vi "InitializeBuffers.vi"(0 "BufferConfig":T1={"Channels"=[], "pretriggerTime_sec"=0.0, "posttriggerTime_sec"=0.0, "BlockSizePerChannel"=0, "SampleRate_Hz"=0.0, "decimation factor"=1, "logDirectory"="", "logPrefix"="", "max files"=0}, 11 "error in (no error)":errorcluster) -> (4 "Buffers":T2={"Channels"=[], "PosttriggerBuffer"=refnum, "PretriggerBuffer"=refnum, "BlockSizePerChannel"=0, " logging semaphore"=refnum, "Log refnum"=refnum, "snapshotBuffer"=refnum, "logDirectory"=path "", "logPrefix"="", "decimation factor"=1, "max files"=0, "SampleRate"=0.0}, 15 "error out":errorcluster)   [LabVIEW 2017, in "BufferLogging.lvlib"]
uses:
  BufferLogging.lvlib
  Buffers.ctl
  BufferConfig.ctl
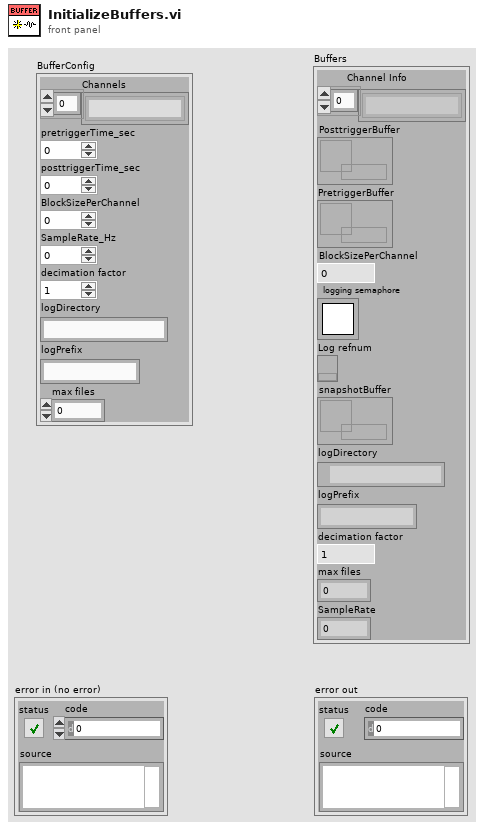
[diagram p1: front panel]
types:
  T1 = typedef "BufferLogging.lvlib/BufferConfig.ctl" = cluster{"Channels":string[], "pretriggerTime_sec":dbl, "posttriggerTime_sec":dbl, "BlockSizePerChannel":i32, "SampleRate_Hz":dbl, "decimation factor":i32, "logDirectory":string, "logPrefix":string, "max files":i32}
  T2 = typedef "BufferLogging.lvlib/Buffers.ctl" = cluster{"Channels":string[], "PosttriggerBuffer":refnum<queue>, "PretriggerBuffer":refnum<queue>, "BlockSizePerChannel":i32, " logging semaphore":T3, "Log refnum":refnum<k34>, "snapshotBuffer":refnum<data-value>, "logDirectory":path, "logPrefix":string, "decimation factor":i32, "max files":i32, "SampleRate":dbl}
  T3 = typedef "Semaphore RefNum" = refnum<k1>
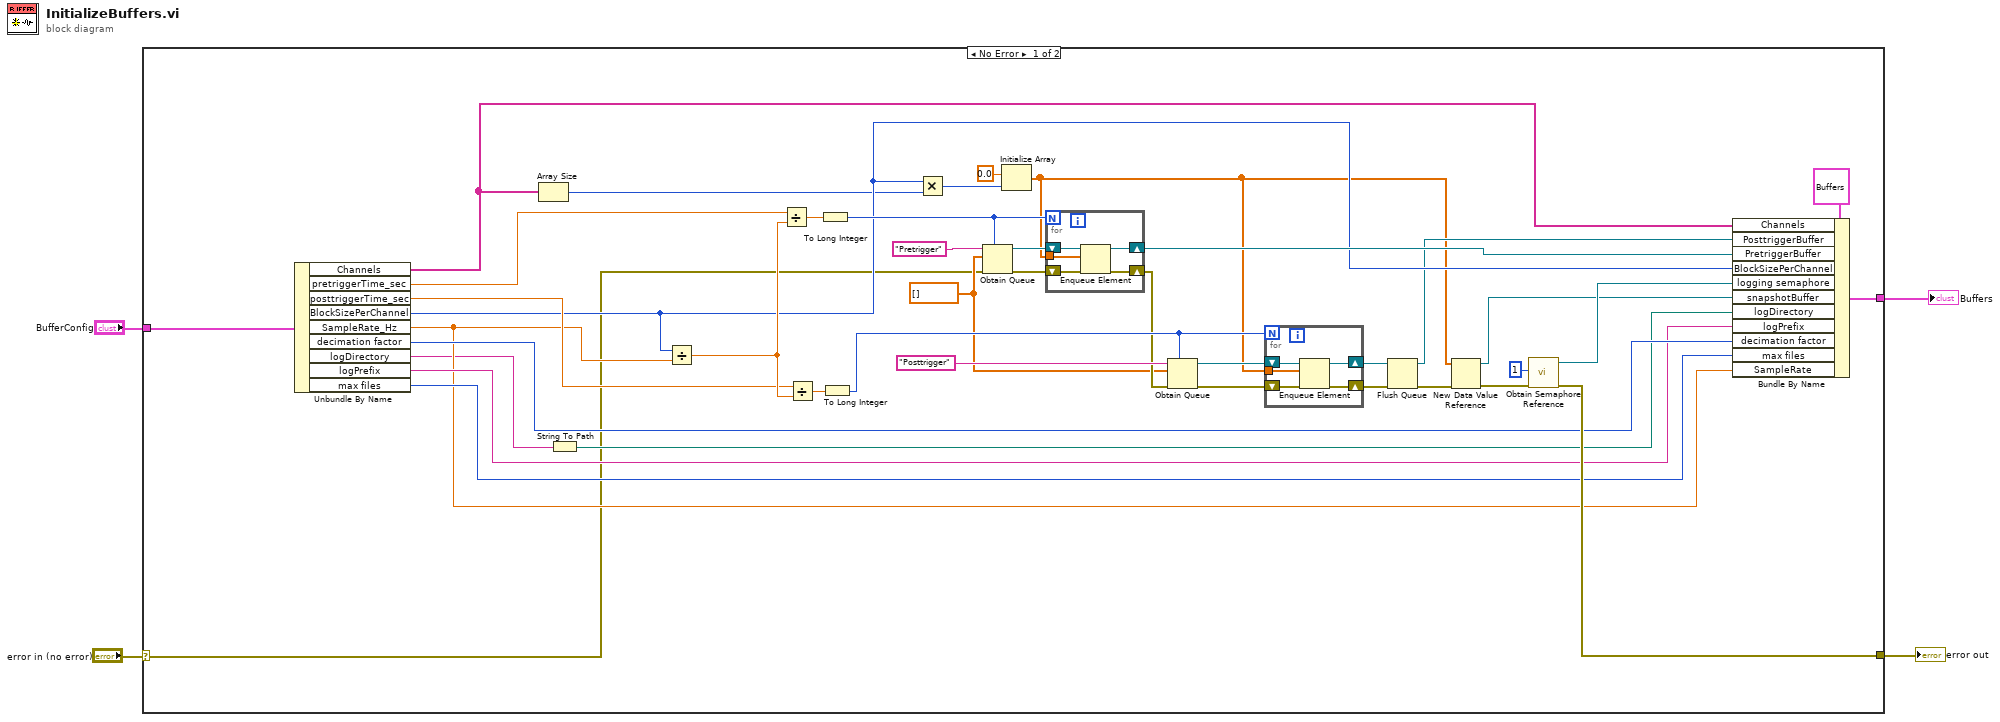
[diagram p0: block diagram]
diagram:
  n1 = case shown="No Error" "error in (no error)" {
    selector: "error in (no error)" -> [w5 w56]
    tunnel: [w31 _] -> w4
    tunnel: [w27 w56] -> w3
    tunnel: "BufferConfig" -> [w26 _]
    frame No Error {
      w18 = sgl[] [] ("Data")
      n2 = Unbundle By Name(w26) -> ("Channels"=w12:string[], "pretriggerTime_sec"=w25:dbl, "posttriggerTime_sec"=w24:dbl, "BlockSizePerChannel"=w22:i32, "SampleRate_Hz"=w8:dbl, "decimation factor"=w11:i32, "logDirectory"=w6:string, "logPrefix"=w10:string, "max files"=w9:i32)
      n3 = Array Size(array=w12) -> (size(s)=w13:i32)
      n4 = String To Path(string=w6) -> (path=w7:path)
      n5 = Divide(x=w22, y=w8) -> (x/y=w43:dbl)
      n6 = Divide(x=w25, y=w43) -> (x/y=w39:dbl)
      n7 = Divide(x=w24, y=w43) -> (x/y=w44:dbl)
      n8 = To Long Integer(number=w39) -> (32bit integer=w40:i32)
      n9 = To Long Integer(number=w44) -> (32bit integer=w45:i32)
      n10 = Multiply(x=w22, y=w13) -> (x*y=w23:i32)
      n11 = Obtain Queue(max queue size (-1, unlimited)=w40, name (unnamed)="Pretrigger", element data type=w18, error in (no error)=w5) -> (queue out=w36:refnum<queue>, error out=w37:errorcluster)  [unwired: 1 in, 1 out]
      n12 = Initialize Array(sgl 0.0 ("element"), w23) -> (w17:sgl[])
      n13 = for {
        N: w40 -> [_]
        tunnel: w17 -> [w53]
        shift-right: [w52] -> w30
        shift-left: w36 -> [w55]
        shift-right: [w51] -> w34
        shift-left: w37 -> [w54]
        n14 = Enqueue Element(queue=w55, element=w53, error in (no error)=w54) -> (queue out=w52:refnum<queue>, error out=w51:errorcluster)  [unwired: 1 in, 1 out]
      }
      n15 = Obtain Queue(max queue size (-1, unlimited)=w45, name (unnamed)="Posttrigger", element data type=w18, error in (no error)=w34) -> (queue out=w41:refnum<queue>, error out=w33:errorcluster)  [unwired: 1 in, 1 out]
      n16 = for {
        N: w45 -> [_]
        tunnel: w17 -> [w48]
        shift-right: [w47] -> w21
        shift-left: w41 -> [w50]
        shift-right: [w46] -> w20
        shift-left: w33 -> [w49]
        n17 = Enqueue Element(queue=w50, element=w48, error in (no error)=w49) -> (queue out=w47:refnum<queue>, error out=w46:errorcluster)  [unwired: 1 in, 1 out]
      }
      n18 = Flush Queue(queue=w21, error in (no error)=w20) -> (queue out=w19:refnum<queue>, error out=w16:errorcluster)  [unwired: 1 out]
      n19 = New Data Value Reference(data value=w17, error in=w16) -> (data value reference=w15:refnum<data-value>, error out=w14:errorcluster)
      n20 = call <vilib>:"Obtain Semaphore Reference.vi"("error in (no error)"=w14, "size (1)"=1) -> ("error out"=w27:errorcluster, "semaphore"=w28:T3)  [unwired: 3 in, 1 out]
      n21 = Bundle By Name(cluster=T2 {"Channels"=[], "PosttriggerBuffer"=refnum, "PretriggerBuffer"=refnum, "BlockSizePerChannel"=0, " logging semaphore"=refnum, "Log refnum"=refnum, "snapshotBuffer"=refnum, "logDirectory"=path "", "logPrefix"="", "decimation factor"=1, "max files"=0, "SampleRate"=0.0} ("Buffers"), "Channels"=w12, "PosttriggerBuffer"=w19, "PretriggerBuffer"=w30, "BlockSizePerChannel"=w22, "logging semaphore"=w28, "snapshotBuffer"=w15, "logDirectory"=w7, "logPrefix"=w10, "decimation factor"=w11, "max files"=w9, "SampleRate"=w8) -> (w31:T2)
    }
    frame Error {
    }
  }
  "error out" <- w3
  "Buffers" <- w4
